vi "Setup State.vi"(8 "error in (no error)":errorcluster, 9 "Setup State (6:Preset)":u16(ring)=6 items=["State 0", "State 1", "State 2", "State 3", "State 4", "State 5", "Preset State"], 10 "Recall/Save (F=Recall)":bool, 11 "VISA Resource Name":refnum<visa-resource-name>) -> (0 "error out":errorcluster, 3 "VISA Resource Name Out":refnum<visa-resource-name>)   [LabVIEW 2020, in "Agilent 34970.lvlib"]
doc: "This VI allows you to save or recall an instrument setup state. You can save a current configuration to states 0-5, or you can recall a setup from states 0-5 or the instrument's preset state."
uses:
  Agilent 34970.lvlib
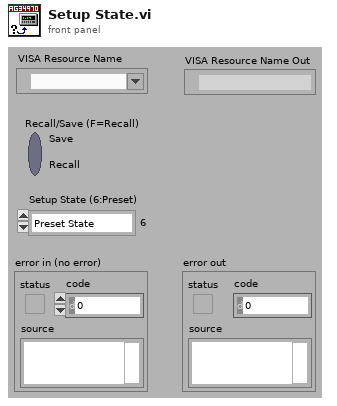
[diagram p1: front panel]
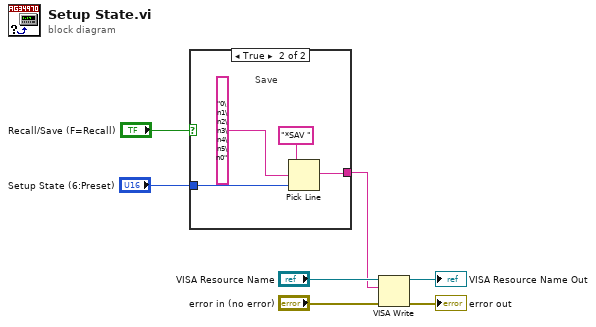
[diagram p0: block diagram]
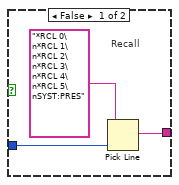
[diagram p2: hidden frame]
diagram:
  n1 = case shown="True" "Recall/Save (F=Recall)" {
    tunnel: "Setup State (6:Preset)" -> [w10 w13]
    tunnel: [w8 w11] -> w3
    frame False {
      # "Recall"
      n2 = Pick Line(multi-line string="*RCL 0\n*RCL 1\n*RCL 2\n*RCL 3\n*RCL 4\n*RCL 5\nSYST:PRES", line index=w10) -> (output string=w8:string)  [unwired: 1 in]
    }
    frame True {
      # "Save"
      n3 = Pick Line(string ("")="*SAV ", multi-line string="0\n1\n2\n3\n4\n5\n0", line index=w13) -> (output string=w11:string)
    }
  }
  n4 = VISA Write(VISA resource name="VISA Resource Name", write buffer=w3, error in (no error)="error in (no error)") -> (VISA resource name out=→"VISA Resource Name Out":refnum<visa-resource-name>, error out=→"error out":errorcluster)  [unwired: 1 out]
